vi "Get Copilot Notifcations Queue Reference.vi"(8 "Error In":errorcluster) -> (0 "Error Out":errorcluster, 3 "Co Pilot Notifications Queue Out":refnum<queue>)   [LabVIEW 2014]
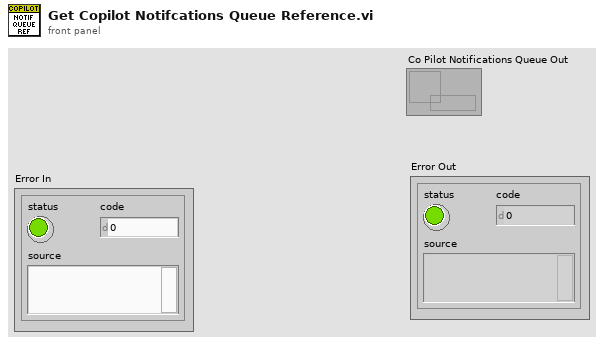
[diagram p1: front panel]
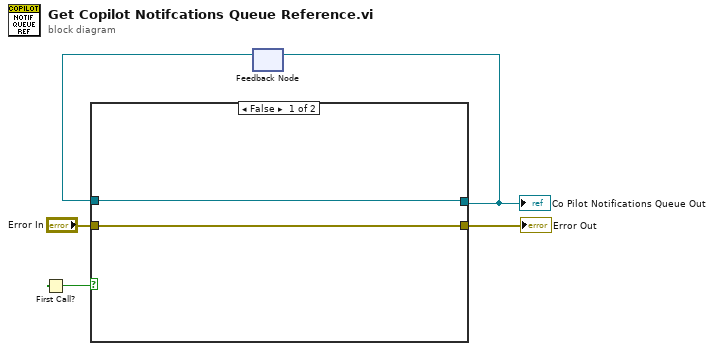
[diagram p0: block diagram]
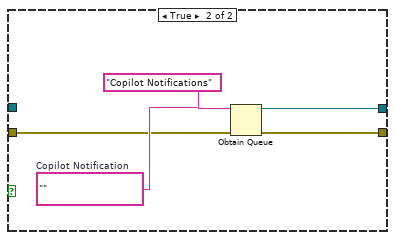
[diagram p2: hidden frame]
diagram:
  n1 = First Call?() -> (First Call?: T/F=w5:bool)
  n2 = feedback #1() -> (w3:refnum<queue>)  [unwired: 1 in]
  n3 = case shown="False" w5 {
    tunnel: [w7 w10] -> w4
    tunnel: w3 -> [w7 _]
    tunnel: "Error In" -> [w6 w9]
    tunnel: [w6 w8] -> w1
    frame False {
    }
    frame True {
      w11 = ""  # Copilot Notification
      n4 = Obtain Queue(name (unnamed)="Copilot Notifications", element data type=w11, error in (no error)=w9) -> (queue out=w10:refnum<queue>, error out=w8:errorcluster)  [unwired: 2 in, 1 out]
    }
  }
  "Error Out" <- w1
  "Co Pilot Notifications Queue Out" <- w4
  n5 = feedback-in #1(w4) -> ()
